vi "Video Toolset Start.vi"(1 "Snapshot Folder":path=path "C:/Users/WET-KORR/Desktop/Screenshots", 2 "Camera Name":string="HD USB Camera") -> ()   [LabVIEW 2010]
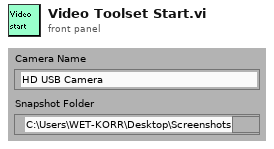
[diagram p1: front panel]
types:
  T1 = enum32{"Bad", "Idle", "Run top level", "Running"}
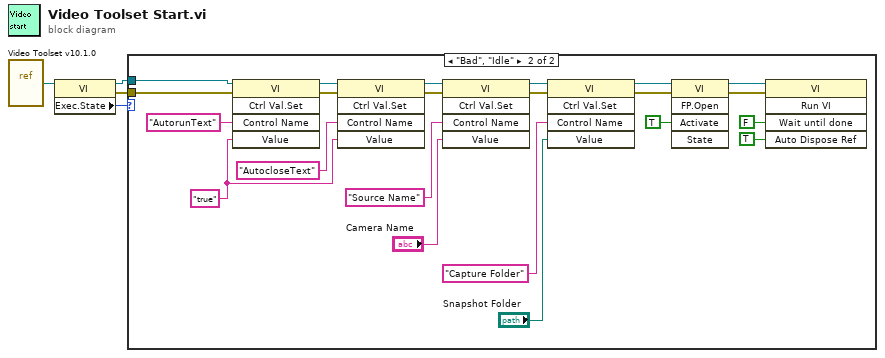
[diagram p0: block diagram]
diagram:
  n1 = vi-ref "Video Toolset v10.1.0.vi"() -> (w4:refnum<vi>)
  n2 = property class="VI"(reference=w4) -> (reference out=w3:refnum<vi>, error out=w1:errorcluster, "Exec.State"=w2:T1)  [unwired: 1 in]
  n3 = case shown="\"Bad\", \"Idle\"" w2 {
    tunnel: w3 -> [_ w6]
    tunnel: w1 -> [_ w5]
    frame Default {
    }
    frame "Bad", "Idle" {
      w9 = "true" ("Control Name")
      n4 = invoke class="VI" method="Ctrl Val.Set"(reference=w6, error in=w5, "Control Name"="AutorunText", "Value"=w9) -> (reference out=w14:refnum<vi>, error out=w13:errorcluster)  [unwired: 1 in, 3 out]
      n5 = invoke class="VI" method="Ctrl Val.Set"(reference=w14, error in=w13, "Control Name"="AutocloseText", "Value"=w9) -> (reference out=w10:refnum<vi>, error out=w11:errorcluster)  [unwired: 1 in, 3 out]
      n6 = invoke class="VI" method="Ctrl Val.Set"(reference=w10, error in=w11, "Control Name"="Source Name", "Value"="Camera Name") -> (reference out=w19:refnum<vi>, error out=w18:errorcluster)  [unwired: 1 in, 3 out]
      n7 = invoke class="VI" method="Ctrl Val.Set"(reference=w19, error in=w18, "Control Name"="Capture Folder", "Value"="Snapshot Folder") -> (reference out=w20:refnum<vi>, error out=w21:errorcluster)  [unwired: 1 in, 3 out]
      n8 = invoke on="Invoke Node" class="VI" method="FP.Open"(reference=w20, error in=w21, "Activate"=TRUE ("Activate?")) -> (reference out=w23:refnum<vi>, error out=w22:errorcluster)  [unwired: 2 in, 3 out]
      n9 = invoke on="Invoke Node" class="VI" method="Run VI"(reference=w23, error in=w22, "Wait until done"=FALSE ("Wait Until Done"), "Auto Dispose Ref"=TRUE ("Auto Dispose Reference")) -> ()  [unwired: 1 in, 5 out]
    }
  }
